vi "FGV Messdaten.vi"(0 "Neue Messwerte":sgl[](array[numeric]), 1 "Rohwerte":sgl[](array[numeric]), 7 "Komponente":u16(ring), 9 "Mittelwerte":i32, 11 "Neuer Zeitstempel":timestamp, 12 "Aktionen":T2) -> (2 "Aktuelle Mittelwerte":sgl[](array[numeric]), 3 "Komponente":u16(ring), 4 "Aktuelle Messwerte":sgl[](array[numeric]), 6 "Messdaten":sgl[][](array[numeric]), 8 "Mittelwertdaten":sgl[][](array[numeric]), 10 "Deviation":sgl[](array[numeric]), 13 "Ausgangs-Cluster":T1, 14 "gemittelter Rohwert":sgl, 15 "Zeitstempeln":timestamp[](array[timestamp]))   [LabVIEW 2020, in "Messdaten.lvlib"]
uses:
  Messdaten.lvlib
  Aktionen FGV Messdaten.ctl
  Rolling Average Daten.ctl
  Seiten/FT-IR/Aktionen EVID-Codes.ctl
  Linearisierung V2/Aktion FGV Rohmesswerte sammeln.ctl
  Seiten/FT-IR/Span/Aktion FGV Span.ctl
  Seiten/FT-IR/FGV FT-IR Aktionen.ctl
  Gewichtung (Stichprobe).ctl
  Allgemein/allgemeine Sub-VIs.lvlib
  Seiten/FT-IR/FT-IR.lvlib
  Linearisierung V2/Linearisierung v2.lvlib
  Seiten/FT-IR/Span/Spanfaktor.lvlib
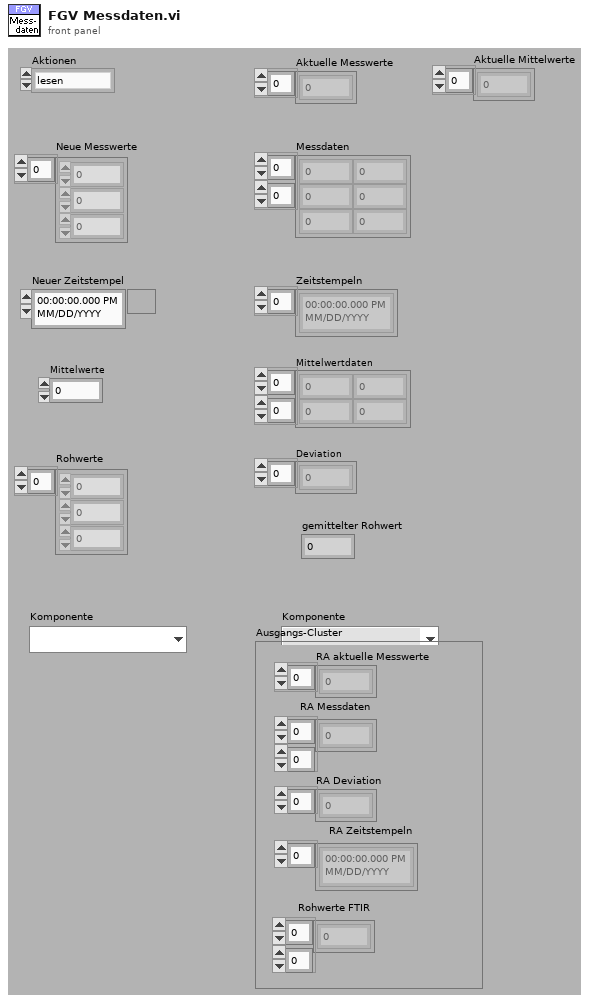
[diagram p1: front panel]
types:
  T1 = typedef "Messdaten.lvlib/Rolling Average Daten.ctl" = cluster{"RA aktuelle Messwerte":sgl[], "RA Messdaten":sgl[][], "RA Deviation":sgl[], "RA Zeitstempeln":timestamp[], "Rohwerte FTIR":sgl[][]}
  T2 = typedef "Messdaten.lvlib/Aktionen FGV Messdaten.ctl" = enum16{"lesen", "schreiben", "löschen", "Mittelwerte", "Komponente"}
  T3 = typedef "FT-IR.lvlib/FGV FT-IR Aktionen.ctl" = enum16{"lesen", "NOG setzen", "NOS setzen", "Initialisieren", "speichern", "ALLES setzen", "FT-IR Spektrum loggen", "Komm Stoppen", "Spektrum LogKonfig"}
  T4 = typedef "FT-IR.lvlib/Spanfaktor.lvlib/Aktion FGV Span.ctl" = enum16{"lesen", "Span", "Seite aktiv", "Offset", "FGV aktualisiert", "Aktualisierung aufheben"}
  T5 = typedef "Linearisierung V2.lvlib/Aktion FGV Rohmesswerte sammeln.ctl" = enum16{"lesen", "schreiben", "löschen", "Sollwert HovaCal"}
  T6 = typedef "FT-IR.lvlib/Aktionen EVID-Codes.ctl" = enum16{"lesen", "setzen", "laden", "speichern", "1Hz/5Hz", "Smoothing", "Rolling Average"}
  T7 = typedef "Messdaten.lvlib/Gewichtung (Stichprobe).ctl" = enum16{"Sample", "Population"}
  T8 = typedef "FT-IR.lvlib/Rolling Average Settings.ctl" = cluster{"Average":u32, "Average via AK:":bool, "Average IAG Software:":bool}
  T9 = typedef "FT-IR.lvlib/1Hz-5Hz Geraet.ctl" = u16
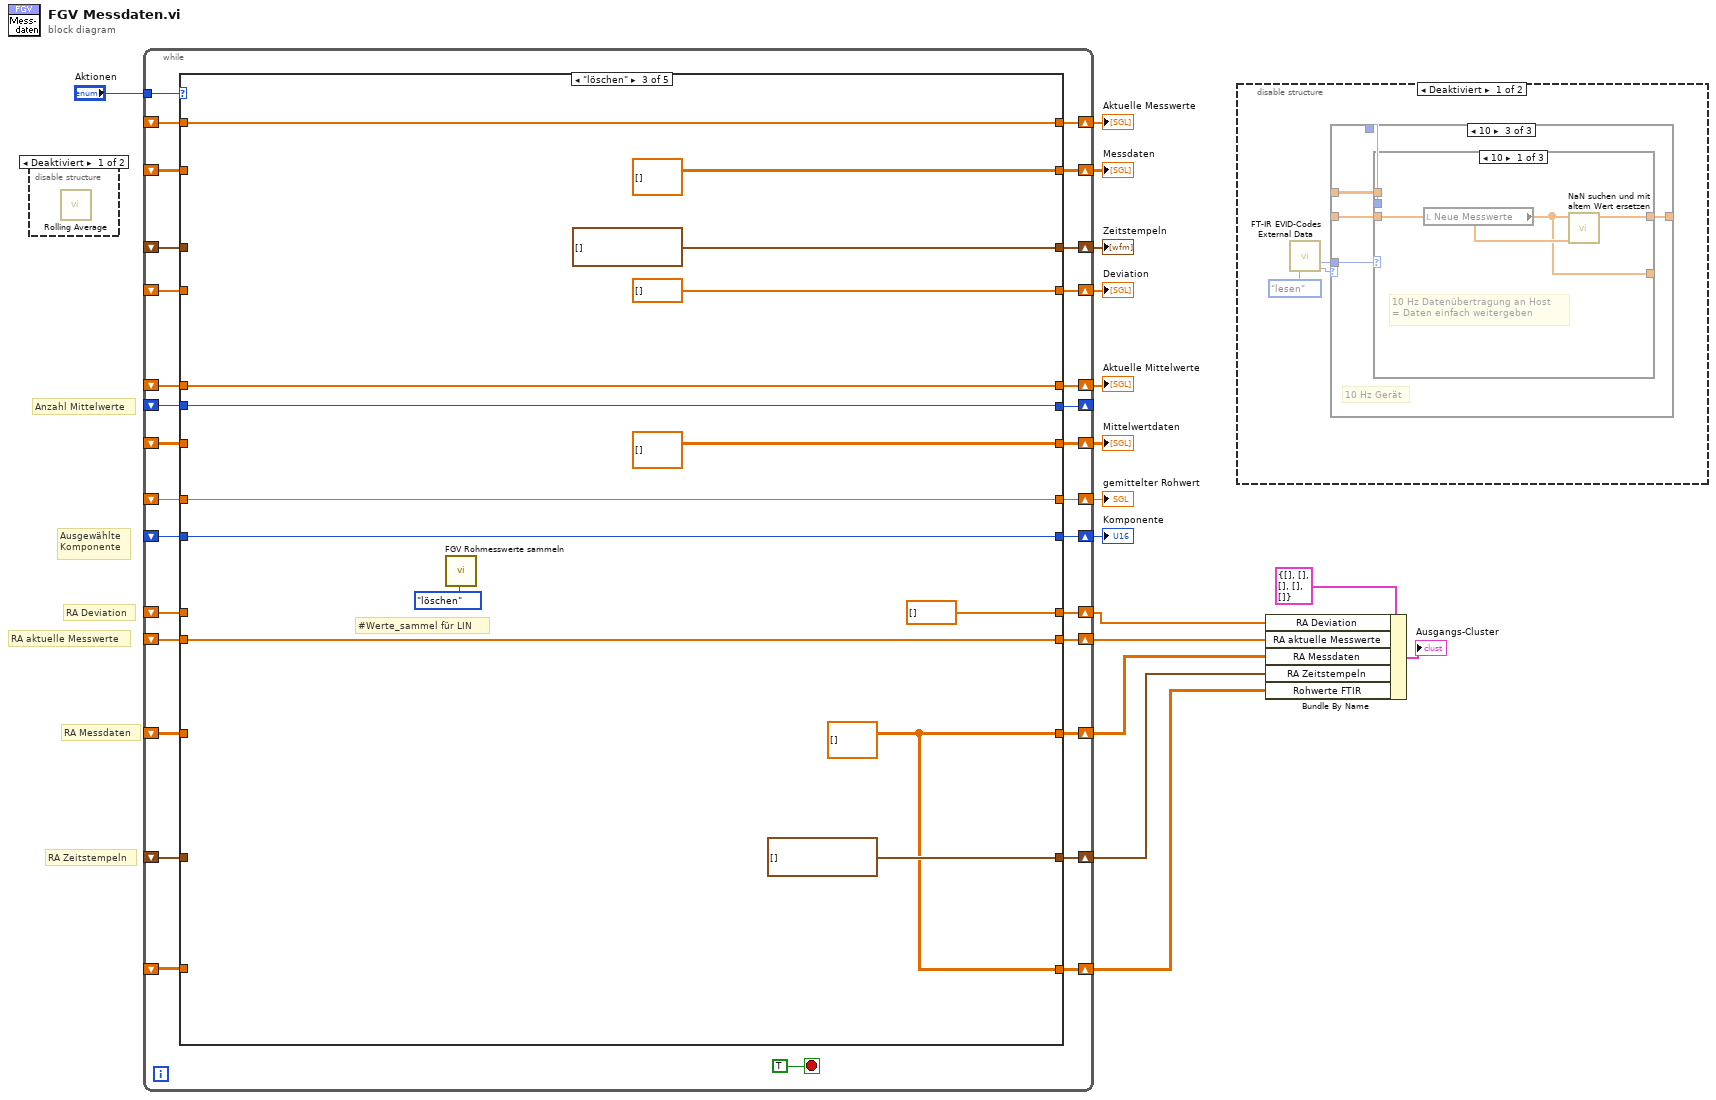
[diagram p0: block diagram]
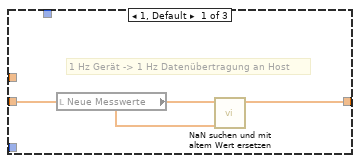
[diagram p2: hidden frame]
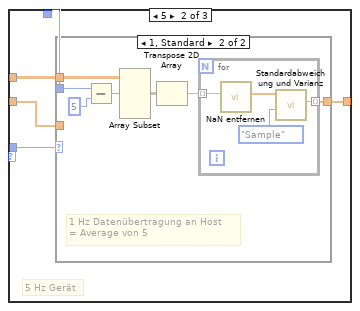
[diagram p3: hidden frame]
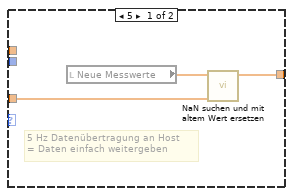
[diagram p4: hidden frame]
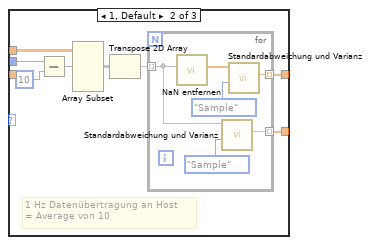
[diagram p5: hidden frame]
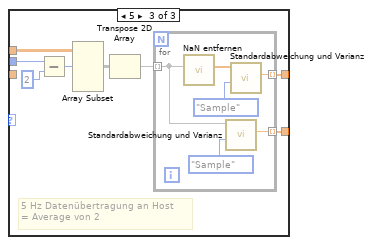
[diagram p6: hidden frame]
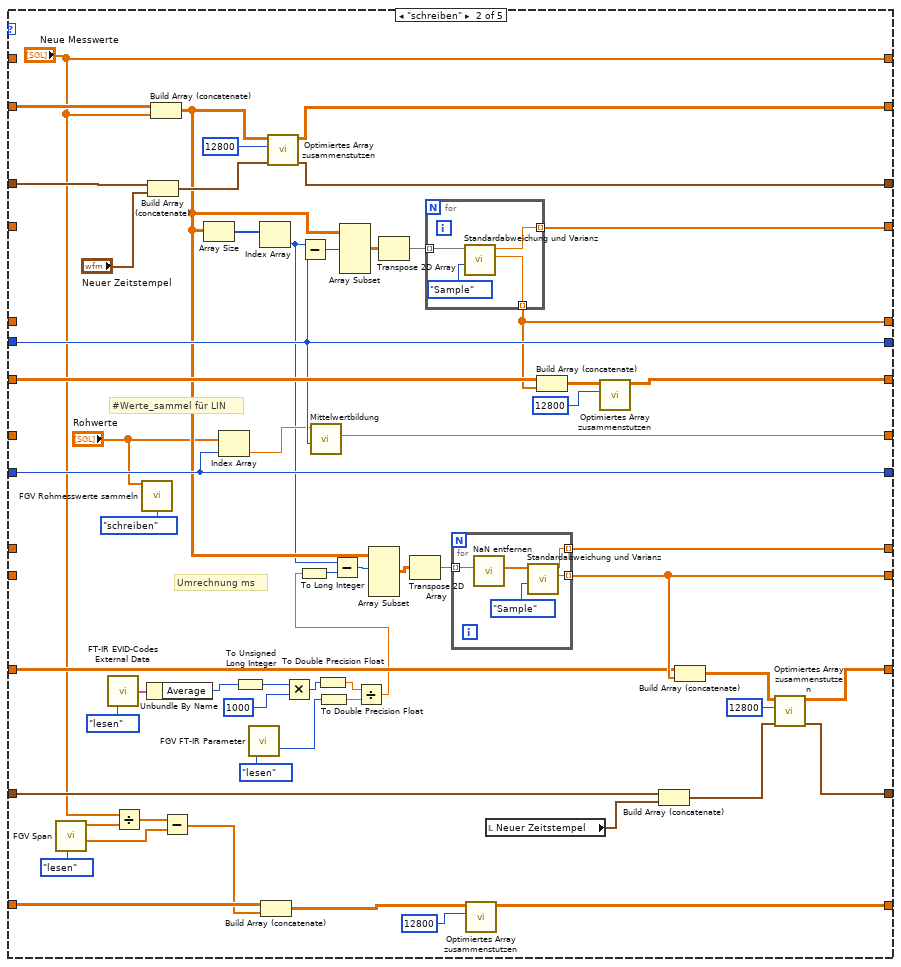
[diagram p10: hidden frame]
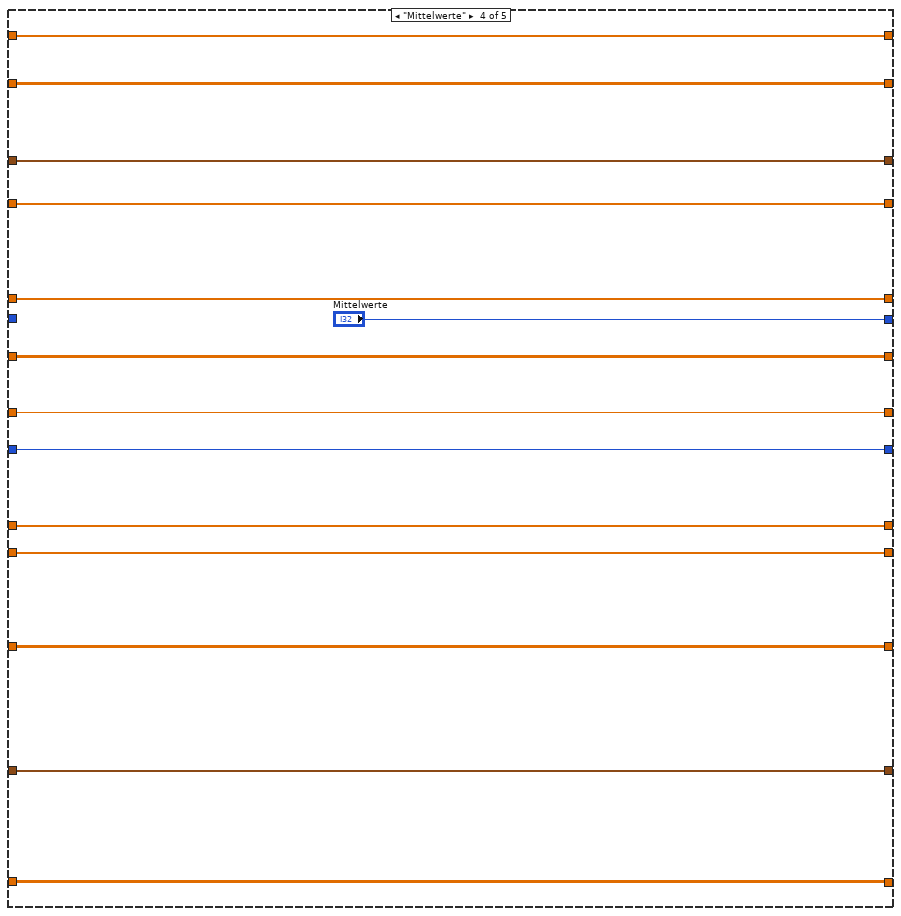
[diagram p11: hidden frame]
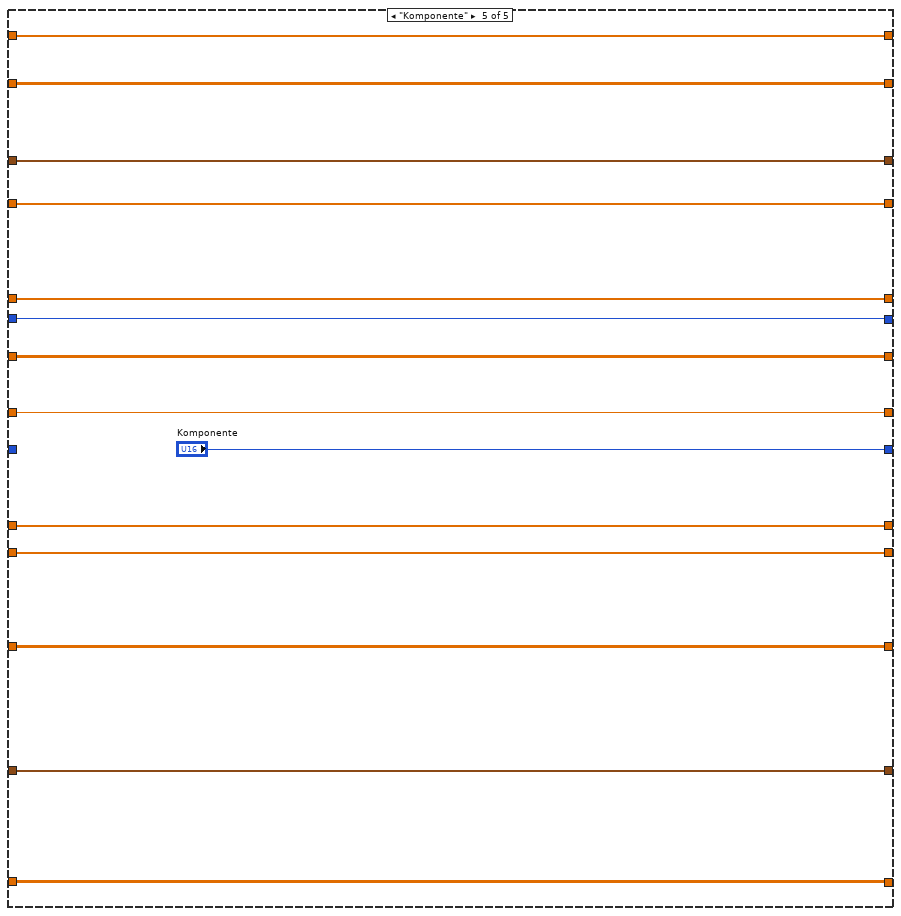
[diagram p12: hidden frame]
diagram:
  # "RA Zeitstempeln"
  # "RA Messdaten"
  # "RA Deviation"
  # "RA aktuelle Messwerte"
  # "Ausgewählte\nKomponente"
  # "Anzahl Mittelwerte"
  n1 = disable-structure shown="Deaktiviert" {
    frame Disabled {
      n2 = call "Rolling Average.vi"() -> ()  [unwired: 10 in, 2 out]
    }
    frame Enabled {
    }
  }
  n3 = while {
    tunnel: "Aktionen" -> [w45]
    shift-right: [w43] -> w15
    shift-left: _ -> [w42]
    shift-right: [w44] -> w14
    shift-left: _ -> [w41]
    shift-right: [w40] -> w13
    shift-left: _ -> [w39]
    shift-right: [w38] -> w12
    shift-left: _ -> [w37]
    shift-right: [w36] -> _
    shift-left: _ -> [w35]
    shift-right: [w34] -> w11
    shift-left: _ -> [w33]
    shift-right: [w32] -> w9
    shift-left: _ -> [w31]
    shift-right: [w30] -> w10
    shift-left: _ -> [w29]
    shift-right: [w28] -> w8
    shift-left: _ -> [w27]
    shift-right: [w26] -> w5
    shift-left: _ -> [w25]
    shift-right: [w23] -> w3
    shift-left: _ -> [w22]
    shift-right: [w24] -> w4
    shift-left: _ -> [w21]
    shift-right: [w20] -> w6
    shift-left: _ -> [w19]
    shift-right: [w18] -> w1
    shift-left: _ -> [w17]
    stop <- TRUE stop-if-true
    n4 = case shown="\"löschen\"" w45 {
      tunnel: [w59 w116 timestamp[] [] w155 w167] -> w44
      tunnel: [w60 w115 sgl[][] [] w156 w166] -> w43
      tunnel: w42 -> [w60 w118 _ w156 w166]
      tunnel: w41 -> [w59 w120 _ w155 w167]
      tunnel: [w58 "Neue Messwerte" w141 w157 w165] -> w40
      tunnel: w39 -> [w58 _ w141 w157 w165]
      tunnel: [w57 w110 sgl[][] [] ("Messdaten") w154 w170] -> w38
      tunnel: w37 -> [w57 w112 _ w154 w170]
      tunnel: [w56 w106 w139 "Mittelwerte" w169] -> w36
      tunnel: w35 -> [w56 w106 w139 _ w169]
      tunnel: [w55 w107 sgl[] [] w152 w168] -> w34
      tunnel: w33 -> [w55 _ _ w152 w168]
      tunnel: [w54 w105 w137 w151 "Komponente"] -> w32
      tunnel: w31 -> [w54 w105 w137 w151 _]
      tunnel: [w53 w103 w136 w150 w164] -> w30
      tunnel: w29 -> [w53 _ w136 w150 w164]
      tunnel: [w52 w100 w135 w149 w163] -> w28
      tunnel: w27 -> [w52 _ w135 w149 w163]
      tunnel: [w51 w91 w134 w148 w162] -> w26
      tunnel: w25 -> [w51 _ w134 w148 w162]
      tunnel: [w49 w90 w130 w146 w160] -> w24
      tunnel: [w48 w89 timestamp[] [] w145 w159] -> w23
      tunnel: w22 -> [w48 w88 _ w145 w159]
      tunnel: w21 -> [w49 w87 _ w146 w160]
      tunnel: [w50 w86 sgl[] [] w147 w161] -> w20
      tunnel: w19 -> [w50 _ _ w147 w161]
      tunnel: [w47 w79 w130 w144 w158] -> w18
      tunnel: w17 -> [w47 w78 _ w144 w158]
      frame "lesen", Default {
      }
      frame "schreiben" {
        # "Umrechnung ms"
        # "#Werte_sammel für LIN"
        n5 = call "FGV Span.vi"("Aktion"=Aktion_FGV_Span."lesen") -> ("Offset"=w63:sgl[], "Span"=w81:sgl[])  [unwired: 7 in, 2 out]
        n6 = call "FT-IR EVID-Codes External Data.vi"("Aktionen"=Aktionen_EVID-Codes."lesen") -> ("Rolling Average Settings"=w85:T8)  [unwired: 9 in, 5 out]
        n7 = Divide(x="Neue Messwerte", y=w81) -> (x/y=w80:sgl[])
        n8 = call "FGV Rohmesswerte sammeln.vi"("Rohwerte"="Rohwerte", "Aktion"=Aktion_FGV_Rohmesswerte_sammeln."schreiben") -> ()  [unwired: 10 in, 4 out]
        n9 = Unbundle By Name(w85) -> ("Average"=w72:u32)
        n10 = Build Array (concatenate)(w120, "Neuer Zeitstempel") -> (w117:timestamp[])
        n11 = Build Array (concatenate)(w118, "Neue Messwerte") -> (w98:sgl[][])
        n12 = Subtract(x=w80, y=w63) -> (x-y=w64:sgl[])
        n13 = Array Size(array=w98) -> (size(s)=w114:i32[])
        n14 = Index Array(array="Rohwerte", index=w105) -> (element=w104:sgl)
        n15 = To Unsigned Long Integer(number=w72) -> (unsigned 32bit integer=w74:u32)
        n16 = call "FGV FT-IR Parameter.vi"("Aktion"=FGV_FT-IR_Aktionen."lesen") -> ("Zykluszeit Messdatenverteiler"=w71:u32)  [unwired: 11 in, 7 out]
        n17 = Index Array(array=w114) -> (element=w97:i32)  [unwired: 1 in]
        n18 = Build Array (concatenate)(w78, w64) -> (w83:sgl[][])
        n19 = call "Optimiertes Array zusammenstutzen.vi"("Zeitstempeln"=w117, "Anzahl Elemente"=12800, "Messdaten"=w98) -> ("Zeitstempeln"=w116:timestamp[], "Messdaten"=w115:sgl[][])  [unwired: 7 in]
        n20 = Multiply(x=w74, y=u32 1000) -> (x*y=w70:u32)
        n21 = Subtract(x=w97, y=w106) -> (x-y=w113:i32)
        n22 = call "Mittelwertbildung.vi"("Anzahl Werte"=w106, "Neuer Wert"=w104) -> ("gemittelter Wert"=w103:sgl)  [unwired: 7 in, 2 out]
        n23 = To Double Precision Float(number=w70) -> (double precision float=w69:dbl)
        n24 = To Double Precision Float(number=w71) -> (double precision float=w68:dbl)
        n25 = Array Subset(array=w98, index (row)=w113) -> (w109:sgl[][])  [unwired: 3 in]
        n26 = Divide(x=w69, y=w68) -> (x/y=w67:dbl)
        n27 = To Long Integer(number=w67) -> (32bit integer=w66:i32)
        n28 = Subtract(x=w97, y=w66) -> (x-y=w61:i32)
        n29 = Array Subset(array=w98, index (row)=w61) -> (w62:sgl[][])  [unwired: 3 in]
        n30 = Transpose 2D Array(2D array=w109) -> (transposed array=w108:sgl[][])
        n31 = Transpose 2D Array(2D array=w62) -> (transposed array=w76:sgl[][])
        n32 = for {
          tunnel: w108 -> [w129] mode=indexing
          tunnel: [w127] -> w100 mode=indexing
          tunnel: [w126] -> w107 mode=indexing
          n33 = call "Standardabweichung und Varianz.vi"("Gewichtung (Stichprobe)"=Gewichtung_(Stichprobe)."Sample", "X"=w129) -> ("Mittelwert"=w127:sgl, "Standardabweichung"=w126:sgl)  [unwired: 7 in, 1 out]
        }
        n34 = for {
          tunnel: w76 -> [w122] mode=indexing
          tunnel: [w124] -> w91 mode=indexing
          tunnel: [w121] -> w86 mode=indexing
          n35 = call "NaN entfernen.vi"("Messdaten"=w122) -> ("Messdaten"=w123:sgl[])  [unwired: 10 in]
          n36 = call "Standardabweichung und Varianz.vi"("Gewichtung (Stichprobe)"=Gewichtung_(Stichprobe)."Sample", "X"=w123) -> ("Mittelwert"=w124:sgl, "Standardabweichung"=w121:sgl)  [unwired: 7 in, 1 out]
        }
        n37 = call "Optimiertes Array zusammenstutzen.vi"("Anzahl Elemente"=12800, "Messdaten"=w83) -> ("Messdaten"=w79:sgl[][])  [unwired: 8 in, 1 out]
        n38 = local read "Neuer Zeitstempel"() -> (w77:timestamp)
        n39 = Build Array (concatenate)(w112, w100) -> (w111:sgl[][])
        n40 = call "Optimiertes Array zusammenstutzen.vi"("Anzahl Elemente"=12800, "Messdaten"=w111) -> ("Messdaten"=w110:sgl[][])  [unwired: 8 in, 1 out]
        n41 = Build Array (concatenate)(w88, w77) -> (w94:timestamp[])
        n42 = Build Array (concatenate)(w87, w91) -> (w93:sgl[][])
        n43 = call "Optimiertes Array zusammenstutzen.vi"("Zeitstempeln"=w94, "Anzahl Elemente"=12800, "Messdaten"=w93) -> ("Zeitstempeln"=w89:timestamp[], "Messdaten"=w90:sgl[][])  [unwired: 7 in]
      }
      frame "löschen" {
        w130 = sgl[][] []
        # "#Werte_sammel für LIN"
        n44 = call "FGV Rohmesswerte sammeln.vi"("Aktion"=Aktion_FGV_Rohmesswerte_sammeln."löschen") -> ()  [unwired: 11 in, 4 out]
      }
      frame "Mittelwerte" {
      }
      frame "Komponente" {
      }
    }
  }
  "Messdaten" <- w15
  "Zeitstempeln" <- w14
  "Aktuelle Messwerte" <- w13
  "Mittelwertdaten" <- w12
  "Deviation" <- w11
  "gemittelter Rohwert" <- w10
  "Komponente" <- w9
  "Aktuelle Mittelwerte" <- w8
  n45 = disable-structure shown="Deaktiviert" {
    frame Disabled {
      n46 = call "FT-IR EVID-Codes External Data.vi"("Aktionen"=Aktionen_EVID-Codes."lesen") -> ("1Hz/5Hz Leitsystem"=w172:T9, "1Hz/5Hz Gerät"=w173:T9)  [unwired: 9 in, 4 out]
      n47 = case shown="10" w173 {
        tunnel: w172 -> [_ w179 w199]
        tunnel: _ -> [_ w182 w200]
        tunnel: _ -> [_ w181 w198]
        tunnel: [w177 w180 w201] -> _
        tunnel: _ -> [w176 w178 w197]
        frame 1, Default {
          # "1 Hz Gerät -> 1 Hz Datenübertragung an Host"
          n48 = local read "Neue Messwerte"() -> (w175:sgl[])
          n49 = call "NaN suchen und mit altem Wert ersetzen.vi"("Alte Messdaten"=w176, "Neue Messdaten"=w175) -> ("Messdaten"=w177:sgl[])  [unwired: 9 in]
        }
        frame 5 {
          # "5 Hz Gerät"
          n50 = case shown="1, Standard" w179 {
            tunnel: w182 -> [_ w189]
            tunnel: w181 -> [_ w188]
            tunnel: [w185 w186] -> w180
            tunnel: w178 -> [w184 _]
            frame 5 {
              # "5 Hz Datenübertragung an Host \n= Daten einfach weitergeben"
              n51 = local read "Neue Messwerte"() -> (w183:sgl[])
              n52 = call "NaN suchen und mit altem Wert ersetzen.vi"("Alte Messdaten"=w184, "Neue Messdaten"=w183) -> ("Messdaten"=w185:sgl[])  [unwired: 9 in]
            }
            frame 1, Default {
              # "1 Hz Datenübertragung an Host \n= Average von 5"
              n53 = Subtract(x=w188, y=5) -> (x-y=w192:i32)
              n54 = Array Subset(array=w189, index (row)=w192) -> (w191:void[][])  [unwired: 3 in]
              n55 = Transpose 2D Array(2D array=w191) -> (transposed array=w190:void[][])
              n56 = for {
                tunnel: w190 -> [w193] mode=indexing
                tunnel: [w195] -> w186 mode=indexing
                n57 = call "NaN entfernen.vi"("Messdaten"=w193) -> ("Messdaten"=w194:sgl[])  [unwired: 10 in]
                n58 = call "Standardabweichung und Varianz.vi"("Gewichtung (Stichprobe)"=Gewichtung_(Stichprobe)."Sample", "X"=w194) -> ("Mittelwert"=w195:sgl)  [unwired: 7 in, 2 out]
              }
            }
          }
        }
        frame 10 {
          # "10 Hz Gerät"
          n59 = case shown="10" w199 {
            tunnel: w200 -> [_ w209 w223]
            tunnel: w198 -> [_ w208 w222]
            tunnel: [w204 w206 w220] -> w201
            tunnel: w197 -> [w203 _ _]
            tunnel: [w202 w205 w219] -> _
            frame 10 {
              # "10 Hz Datenübertragung an Host \n= Daten einfach weitergeben"
              n60 = local read "Neue Messwerte"() -> (w202:sgl[])
              n61 = call "NaN suchen und mit altem Wert ersetzen.vi"("Alte Messdaten"=w203, "Neue Messdaten"=w202) -> ("Messdaten"=w204:sgl[])  [unwired: 9 in]
            }
            frame 1, Default {
              # "1 Hz Datenübertragung an Host \n= Average von 10"
              n62 = Subtract(x=w208, y=10) -> (x-y=w212:i32)
              n63 = Array Subset(array=w209, index (row)=w212) -> (w211:void[][])  [unwired: 3 in]
              n64 = Transpose 2D Array(2D array=w211) -> (transposed array=w210:void[][])
              n65 = for {
                tunnel: w210 -> [w214] mode=indexing
                tunnel: [w217] -> w206 mode=indexing
                tunnel: [w213] -> w205 mode=indexing
                n66 = call "NaN entfernen.vi"("Messdaten"=w214) -> ("Messdaten"=w216:sgl[])  [unwired: 10 in]
                n67 = call "Standardabweichung und Varianz.vi"("Gewichtung (Stichprobe)"=Gewichtung_(Stichprobe)."Sample", "X"=w214) -> ("Mittelwert"=w213:sgl)  [unwired: 7 in, 2 out]
                n68 = call "Standardabweichung und Varianz.vi"("Gewichtung (Stichprobe)"=Gewichtung_(Stichprobe)."Sample", "X"=w216) -> ("Mittelwert"=w217:sgl)  [unwired: 7 in, 2 out]
              }
            }
            frame 5 {
              # "5 Hz Datenübertragung an Host \n= Average von 2"
              n69 = Subtract(x=w222, y=2) -> (x-y=w226:i32)
              n70 = Array Subset(array=w223, index (row)=w226) -> (w225:void[][])  [unwired: 3 in]
              n71 = Transpose 2D Array(2D array=w225) -> (transposed array=w224:void[][])
              n72 = for {
                tunnel: w224 -> [w228] mode=indexing
                tunnel: [w231] -> w220 mode=indexing
                tunnel: [w227] -> w219 mode=indexing
                n73 = call "NaN entfernen.vi"("Messdaten"=w228) -> ("Messdaten"=w230:sgl[])  [unwired: 10 in]
                n74 = call "Standardabweichung und Varianz.vi"("Gewichtung (Stichprobe)"=Gewichtung_(Stichprobe)."Sample", "X"=w228) -> ("Mittelwert"=w227:sgl)  [unwired: 7 in, 2 out]
                n75 = call "Standardabweichung und Varianz.vi"("Gewichtung (Stichprobe)"=Gewichtung_(Stichprobe)."Sample", "X"=w230) -> ("Mittelwert"=w231:sgl)  [unwired: 7 in, 2 out]
              }
            }
          }
        }
      }
    }
    frame Enabled {
    }
  }
  n76 = Bundle By Name(cluster=T1 {"RA aktuelle Messwerte"=[], "RA Messdaten"=[], "RA Deviation"=[], "RA Zeitstempeln"=[], "Rohwerte FTIR"=[]} ("Rolling Average Daten"), "RA Deviation"=w6, "RA aktuelle Messwerte"=w5, "RA Messdaten"=w4, "RA Zeitstempeln"=w3, "Rohwerte FTIR"=w1) -> (→"Ausgangs-Cluster":T1)
